vi "Create Map.vi"(8 "error in (no error)":errorcluster, 11 "ATM Data":T1={"UI Refs"={"Right Buttons"=refnum, "Left Buttons"=refnum, "User Input"=refnum, "ATM Messages"=refnum, "Left Menu"=refnum, "Right Menu"=refnum, "Enter"=refnum}, "Map"={}, "Login Valid?"=FALSE, "Queue Message"=refnum, "State"=enum."None", "User"={"Pin"="", "First Name"="", "Last Name"="", "Balance"=0.0, "Login Valid?"=FALSE}, "Main States"={"Message"="Initialize", "Data"=variant}}) -> (0 "error out":errorcluster, 3 "ATM Data Out":T1={"UI Refs"={"Right Buttons"=refnum, "Left Buttons"=refnum, "User Input"=refnum, "ATM Messages"=refnum, "Left Menu"=refnum, "Right Menu"=refnum, "Enter"=refnum}, "Map"={}, "Login Valid?"=FALSE, "Queue Message"=refnum, "State"=enum."None", "User"={"Pin"="", "First Name"="", "Last Name"="", "Balance"=0.0, "Login Valid?"=FALSE}, "Main States"={"Message"="Initialize", "Data"=variant}})   [LabVIEW 2020, in "ATM Machine.lvlib"]
uses:
  ATM Machine.lvlib
  Cluster - ATM Machine Data.ctl
  Users/khemr/OneDrive/Desktop/Labview Training/CLD/New ATM_KR/ATM Machine/Cluster - Message Cluster.ctl
  Enum - ATM States.ctl
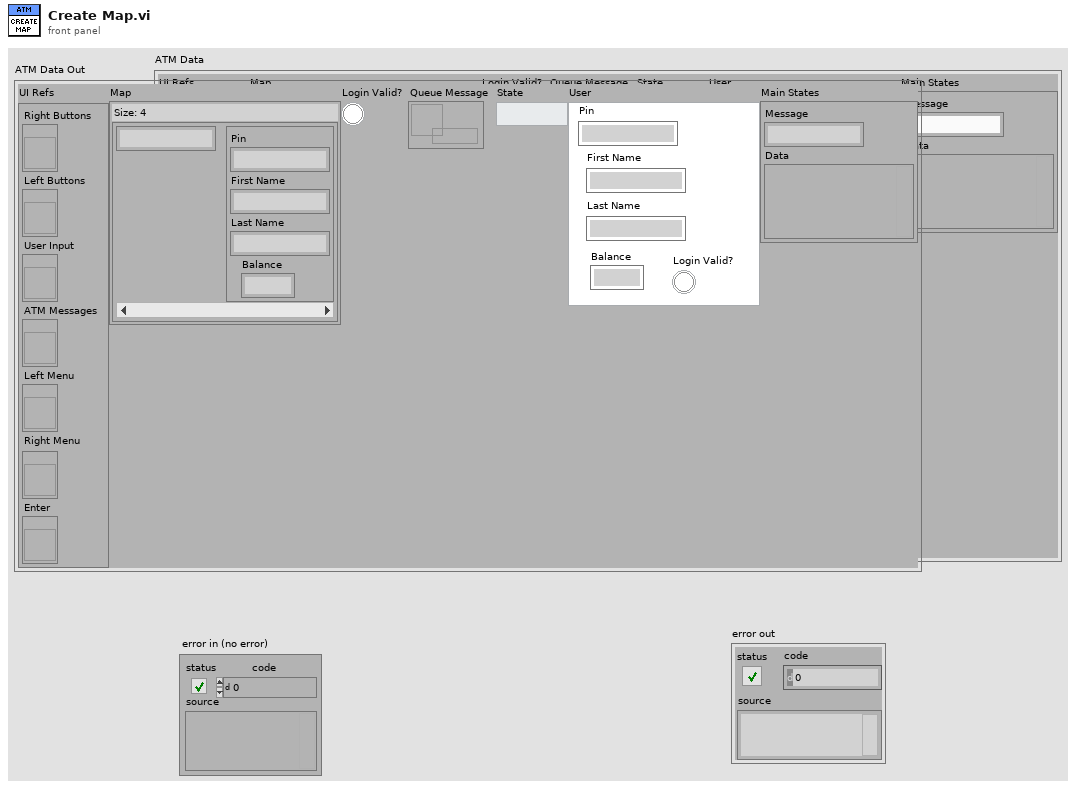
[diagram p1: front panel]
types:
  T1 = typedef "ATM Machine.lvlib/Cluster - ATM Machine Data.ctl" = cluster{"UI Refs":cluster{"Right Buttons":refnum<vi>, "Left Buttons":refnum<vi>, "User Input":refnum<vi>, "ATM Messages":refnum<vi>, "Left Menu":refnum<vi>, "Right Menu":refnum<vi>, "Enter":refnum<vi>}, "Map":map{string, cluster{"Pin":string, "First Name":string, "Last Name":string, "Balance":dbl}}, "Login Valid?":bool, "Queue Message":refnum<queue>, "State":T2, "User":cluster{"Pin":string, "First Name":string, "Last Name":string, "Balance":dbl, "Login Valid?":bool}, "Main States":cluster{"Message":string, "Data":variant}}
  T2 = typedef "ATM Machine.lvlib/Enum - ATM States.ctl" = enum16{"None", "Deposit", "Withdraw", "Card Inserted", "Balance Inquiry", "Return Card and Terminate", "Fast Cash"}
  T3 = map{string, cluster{"Pin":string, "First Name":string, "Last Name":string, "Balance":dbl}}
  T4 = cluster{"Pin":string, "First Name":string, "Last Name":string, "Balance":dbl}
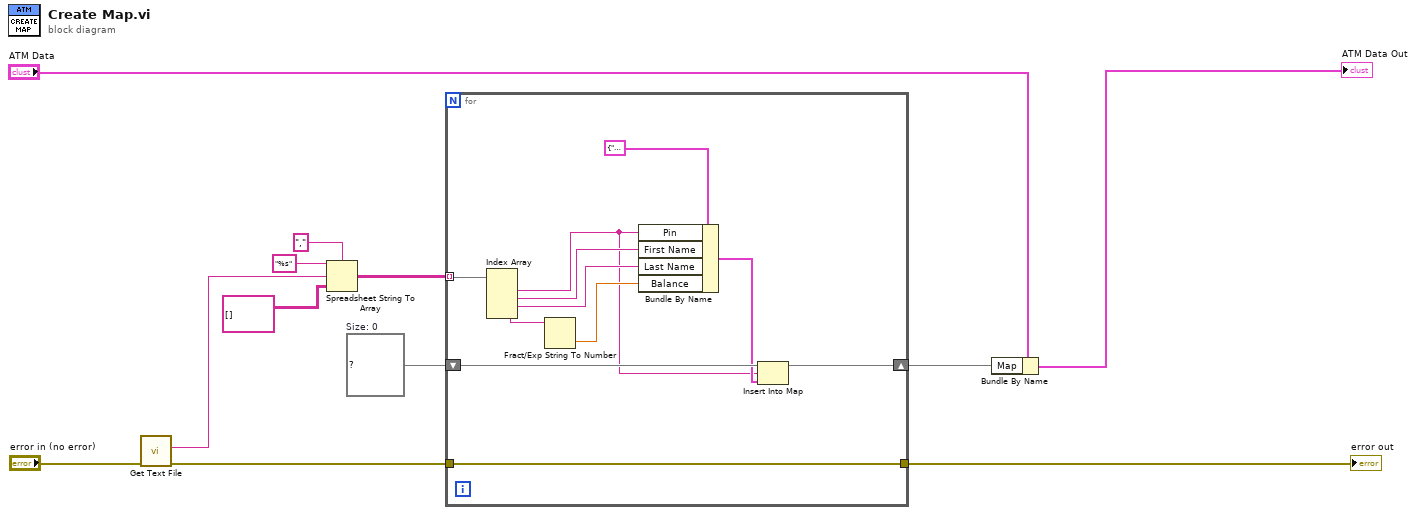
[diagram p0: block diagram]
diagram:
  w4 = T3 {}  # Size: 0
  n1 = call "Get Text File.vi"("error in (no error)"="error in (no error)") -> ("error out"=w6:errorcluster, "File Out"=w5:string)  [unwired: 9 in]
  n2 = Spreadsheet String To Array(delimiter (Tab)=",", format string="%s", spreadsheet string=w5, array type (2D Dbl)=string[][] []) -> (array=w9:string[][])
  n3 = for {
    tunnel: w9 -> [w20] mode=indexing
    shift-right: [w22] -> w2
    shift-left: w4 -> [w23]
    tunnel: [w21] -> w8
    tunnel: w6 -> [w21]
    n4 = Index Array(array=w20) -> (element #1=w13:string, element #2=w16:string, element #3=w15:string, element #4=w19:string)  [unwired: 4 in]
    n5 = Fract/Exp String To Number(string=w19) -> (number=w14:dbl)  [unwired: 3 in, 1 out]
    n6 = Bundle By Name(cluster=T4 {"Pin"="", "First Name"="", "Last Name"="", "Balance"=0.0}, "Pin"=w13, "First Name"=w16, "Last Name"=w15, "Balance"=w14) -> (w18:T4)
    n7 = Insert Into Map(map in=w23, key=w13, value=w18) -> (map out=w22:T3)  [unwired: 2 out]
  }
  "error out" <- w8
  n8 = Bundle By Name(cluster="ATM Data", "Map"=w2) -> (→"ATM Data Out":T1)
